vi "OnDemandWaveformDataBroadcast_Parse.vi"(8 "error in (no error)":errorcluster, 11 "message":variant) -> (0 "error out":errorcluster, 2 "on demand waveform":T1)   [LabVIEW 2017, in "EmsaAcquisition.lvlib"]
uses:
  <vilib>/addons/InsightCM/Devices/Shared/Emsa/EmsaAcquisition/EmsaAcquisition.lvlib
  <vilib>/addons/InsightCM/Devices/Shared/Emsa/EmsaAcquisition/controls/OnDemandWaveformData.ctl
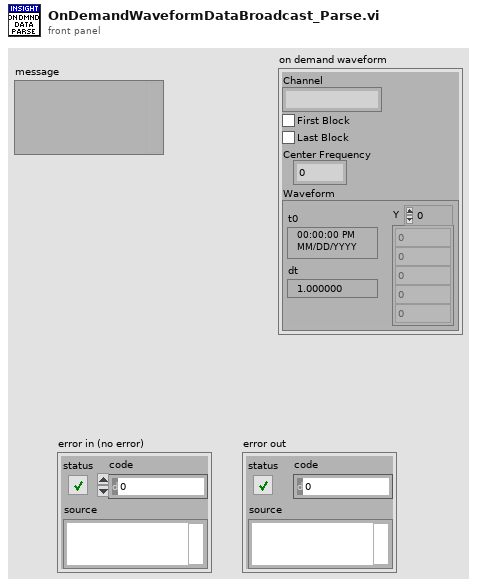
[diagram p1: front panel]
types:
  T1 = typedef "EmsaAcquisition.lvlib/OnDemandWaveformData.ctl" = cluster{"Channel":string, "First Block":bool, "Last Block":bool, "Center Frequency":dbl, "Waveform":waveform(dbl)}
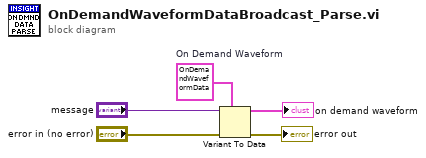
[diagram p0: block diagram]
diagram:
  w5 = T1 {"Channel"="", "First Block"=FALSE, "Last Block"=FALSE, "Center Frequency"=0.0, "Waveform"={"t0"=timestamp(0 s since 1904-01-01), "dt"=1.0, "Y"=[]}}  # On Demand Waveform
  n1 = Variant To Data(error in="error in (no error)", type=w5, Variant="message") -> (data=→"on demand waveform":T1, error out=→"error out":errorcluster)
